vi "fileIO.vi"(0 "access (0:read/write)":enum16{"read/write", "read-only", "write-only"}(ring), 1 "operation (0:open)":T1(ring), 2 "file path (use dialog)":path, 3 "text":string) -> ()   [LabVIEW 2013]
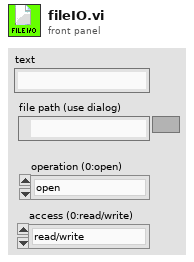
[diagram p1: front panel]
types:
  T1 = enum16{"open", "replace", "create", "open or create", "replace or create", "replace or create with confirmation"}
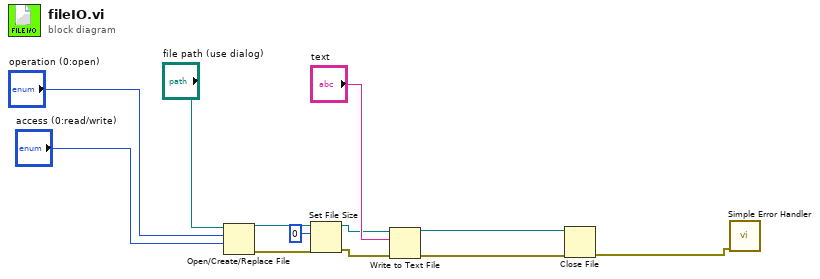
[diagram p0: block diagram]
diagram:
  n1 = Open/Create/Replace File(file path (use dialog)="file path (use dialog)", operation (0:open)="operation (0:open)", access (0:read/write)="access (0:read/write)") -> (refnum out=w5:refnum<file>, error out=w4:errorcluster)  [unwired: 3 in, 1 out]
  n2 = Set File Size(4:w4, 6:i64 0 ("size (in bytes)"), 7:w5) -> (0:w3:errorcluster, 3:w2:refnum<file>)
  n3 = Write to Text File(file (use dialog)=w2, text="text", error in=w3) -> (refnum out=w11:refnum<file>, error out=w10:errorcluster)  [unwired: 1 in, 1 out]
  n4 = Close File(refnum=w11, error in=w10) -> (error out=w12:errorcluster)  [unwired: 1 out]
  n5 = call <vilib>:"Simple Error Handler.vi"("error in (no error)"=w12) -> ()  [unwired: 4 in, 5 out]
